vi "va-cam0#B1A2.vi"(0 "Image In":T2, 1 "Image Dst":T2, 2 "ROI Descriptor (Cent)":T1={"Global Rectangle"=[1001, 801, 1479, 1278], "Contours"=[{"ID"=enum."External", "Type"=7, "Coordinates"=[1239, 1039, 28, 238, 0, 0]}]} {"Contours"."Type" items=["No Selection", "Point", "Line", "Rectangle", "Oval", "Polygon", "Freehand Region", "Annulus", "Unused2", "Unused3", "Broken Line", "Freehand Line", "Rotated Rectangle"]}, 3 "ROI Descriptor (cir_pro_raw)":T1={"Global Rectangle"=[1854, 674, 1995, 880], "Contours"=[{"ID"=enum."External", "Type"=7, "Coordinates"=[1997, 735, 91, 143, 155136, 267537]}]} {"Contours"."Type" items=["No Selection", "Point", "Line", "Rectangle", "Oval", "Polygon", "Freehand Region", "Annulus", "Unused2", "Unused3", "Broken Line", "Freehand Line", "Rotated Rectangle"]}, 7 "error in":errorcluster) -> (19 "Caliper Results (angle_Cent_pro_fine)":sgl[][](array[numeric]) format="%.2f", 20 "Image Out":T2, 21 "Fitted Circle (Cent)":T4 {"Average SNR (dB)" format="%.2f"; "Average Strength" format="%.2f"; "Roundness (Real-World)" format="%.2f"; "Radius (Real-World)" format="%.2f"; "Center (Real-World)"."Y" format="%.2f"; "Center (Real-World)"."X" format="%.2f"; "Radius (Pixels)" format="%.2f"; "Center (Pixels)"."Y" format="%.2f"; "Center (Pixels)"."X" format="%.2f"}, 22 "Fitted Circle (cir_pro_Fine)":T4 {"Average SNR (dB)" format="%.2f"; "Average Strength" format="%.2f"; "Roundness (Real-World)" format="%.2f"; "Radius (Real-World)" format="%.2f"; "Center (Real-World)"."Y" format="%.2f"; "Center (Real-World)"."X" format="%.2f"; "Radius (Pixels)" format="%.2f"; "Center (Pixels)"."Y" format="%.2f"; "Center (Pixels)"."X" format="%.2f"}, 23 "Edge Information (edge_Find_SlotSidesLo)":T3[](array[typedef]) {"Distance (Real-World)" format="%.2f"; "Location (Real-World)"."Y" format="%.2g"; "Location (Real-World)"."X" format="%.2f"; "Noise" format="%.2f"; "Location (Pixel)"."Y" format="%.2g"; "Location (Pixel)"."X" format="%.2f"; "Strength" format="%.2f"; "Distance (Pixel)" format="%.2f"}, 26 "Edge Information (edge_Find_SlotSidesHi)":T3[](array[typedef]) {"Distance (Real-World)" format="%.2f"; "Location (Real-World)"."Y" format="%.2g"; "Location (Real-World)"."X" format="%.2f"; "Noise" format="%.2f"; "Location (Pixel)"."Y" format="%.2g"; "Location (Pixel)"."X" format="%.2f"; "Strength" format="%.2f"; "Distance (Pixel)" format="%.2f"}, 27 "error out":errorcluster)   [LabVIEW 2018]
doc: "Creates, edits, and runs vision algorithms using NI Vision Assistant.\n\nWhen you place this Express VI on the block diagram, NI Vision Assistant launches. Create an algorithm using the Vision Assistant processing functions. After you create an algorithm, you can select the controls and indicators that you want to be able to programmatically set in LabVIEW. Double-click the Vision Assistant Express VI to edit the algorithm."
uses:
  <vilib>/vision/Image Controls.llb/IMAQ Image.ctl
  <vilib>/vision/Measure.llb/Edge New.ctl
  <vilib>/vision/Measure.llb/Edge Options.ctl
  <vilib>/vision/Measure.llb/Edge Polarity.ctl
  <vilib>/vision/NI_Vision_Development_Module.lvlib
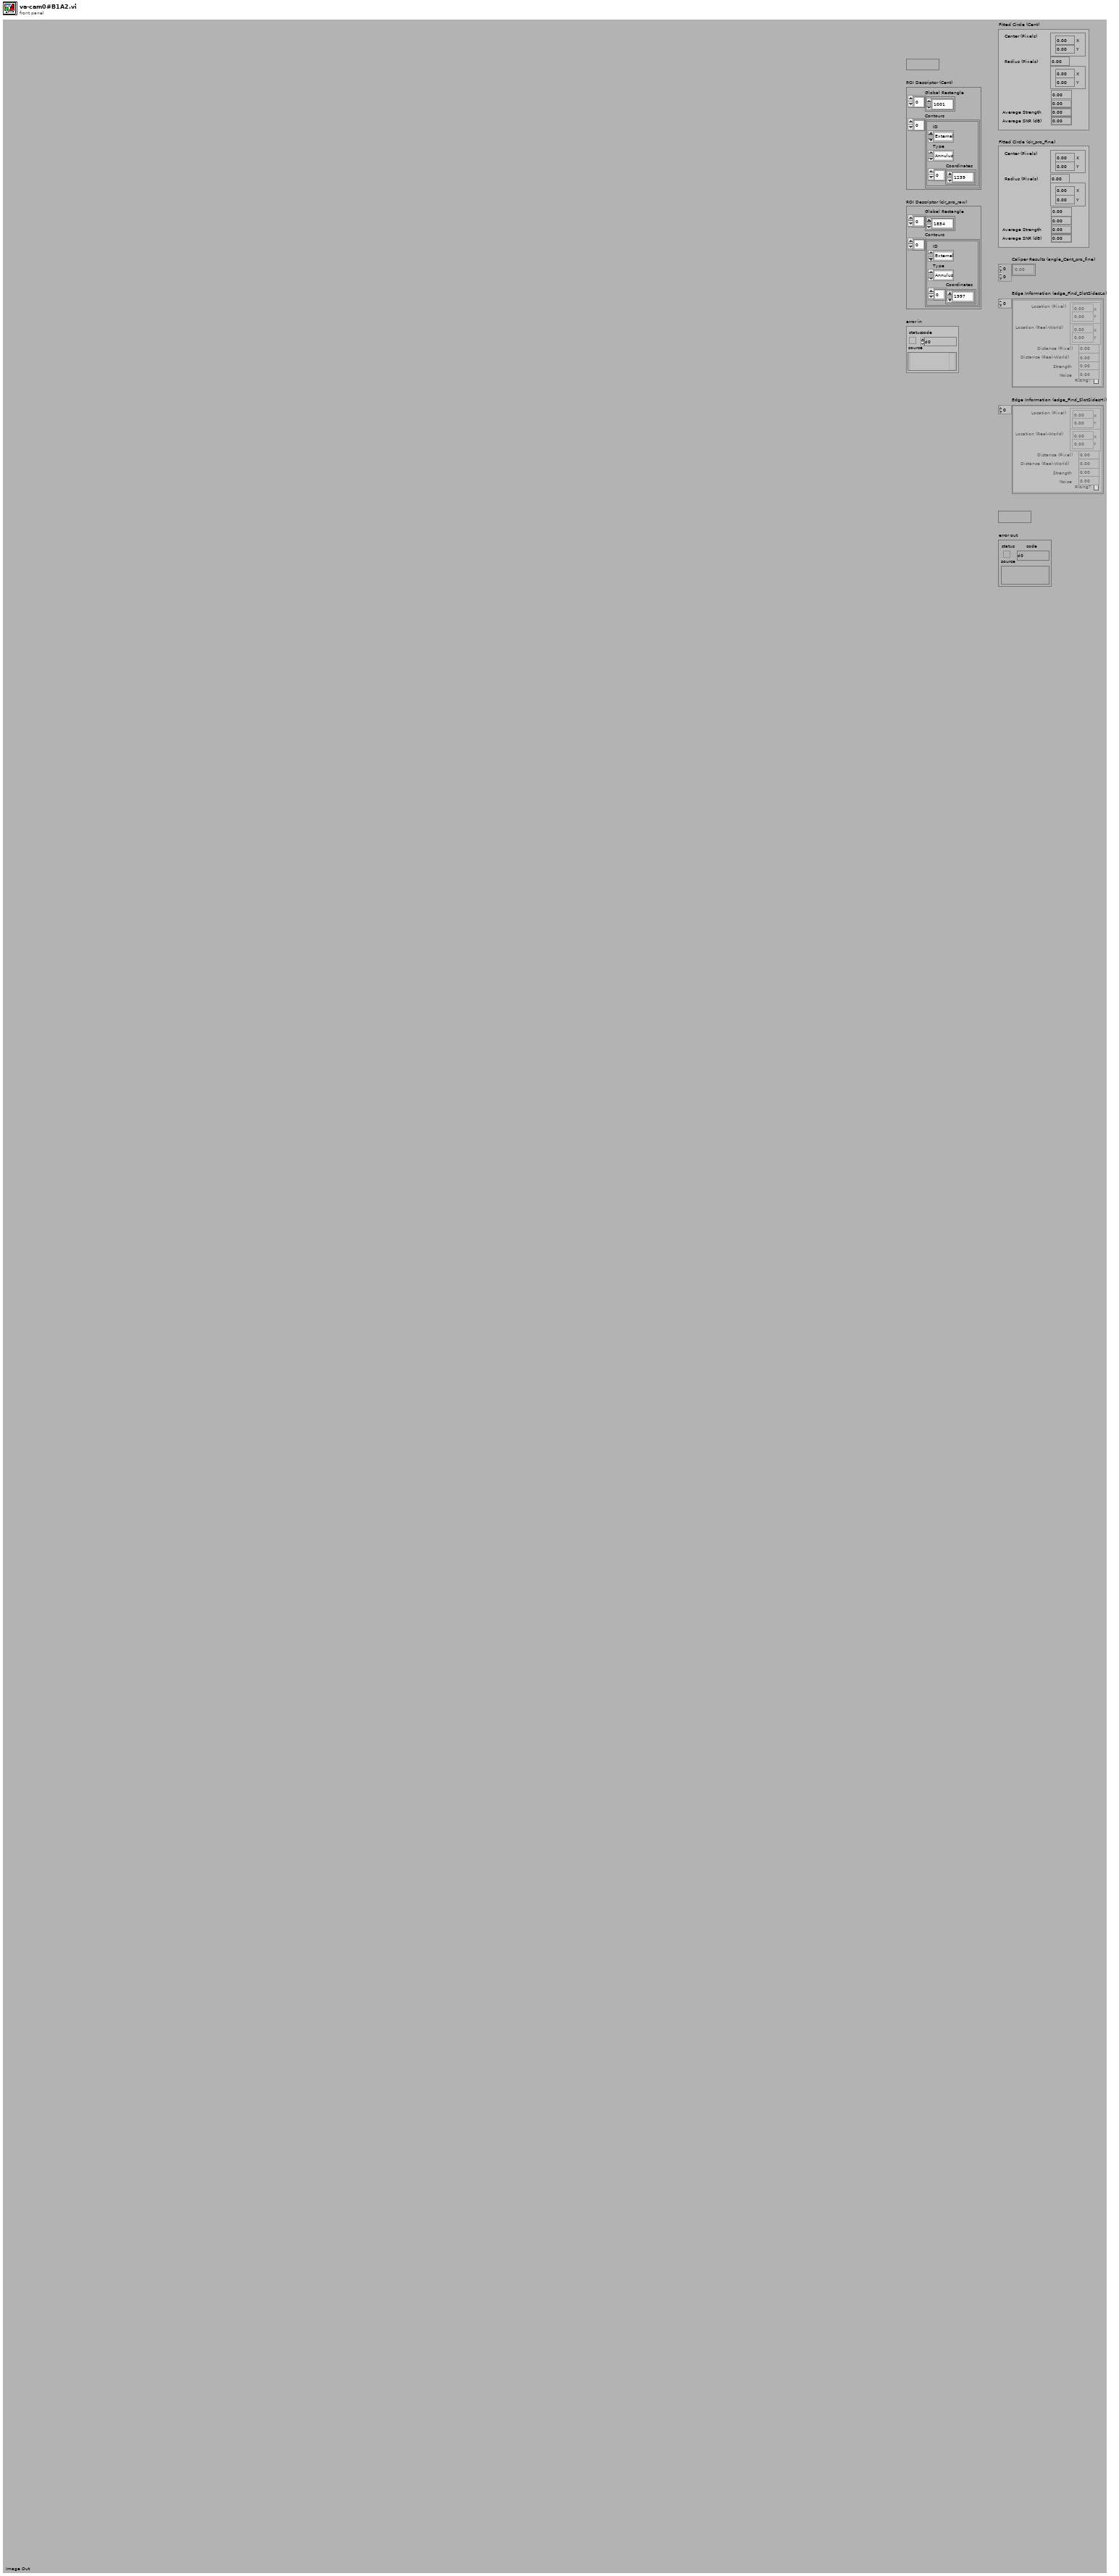
[diagram p1: front panel]
types:
  T1 = cluster{"Global Rectangle":i32[], "Contours":cluster{"ID":enum32{"External", "Internal"}, "Type":u32, "Coordinates":i32[]}[]}
  T2 = typedef "IMAQ Image.ctl" = refnum<image>
  T3 = typedef "Edge New.ctl" = cluster{"Location (Pixel)":cluster{"X":sgl, "Y":sgl}, "Location (Real-World)":cluster{"X":sgl, "Y":sgl}, "Distance (Pixel)":dbl, "Distance (Real-World)":dbl, "Strength":dbl, "Noise":dbl, "Rising?":bool}
  T4 = cluster{"Center (Pixels)":cluster{"X":sgl, "Y":sgl}, "Radius (Pixels)":dbl, "Center (Real-World)":cluster{"X":sgl, "Y":sgl}, "Radius (Real-World)":dbl, "Roundness (Real-World)":dbl, "Average Strength":dbl, "Average SNR (dB)":dbl}
  T5 = cluster{"Edge Polarity":u32, "Kernel Size":u32, "Width":u32, "Minimum Edge Strength":sgl, "Interpolation Type":enum32{"Zero Order", "Bilinear", "Quadratic", "Cubic", "Bilinear Fixed"}, "Data Processing Method":enum32{"Average", "Median"}}
  T6 = enum16{"Get First Edge", "Get First + Last Edge", "Get All Edges", "Get Best Edge"}
  T7 = cluster{"Origin":cluster{"X":sgl, "Y":sgl}, "Angle (deg)":sgl, "Axis Reference":u32}
  T8 = enum16{"Reset", "Update Coordinate System", "Get Coordinate System"}
  T9 = enum16{"Horizontal Motion", "Vertical Motion", "Horizontal and Vertical Motion", "Horizontal, Vertical and Angular Motion"}
  T10 = cluster{"Feature":u32, "Points IDs":cluster{"GUID":string, "Index":i32}[]}[]
  T11 = typedef "Edge Options.ctl" = cluster{"Edge Polarity":T12, "Kernel Size":u32, "Width":u32, "Minimum Edge Strength":sgl, "Interpolation Type":enum32{"Zero Order", "Bilinear", "Quadratic", "Cubic", "Bilinear Fixed"}, "Data Processing Method":enum32{"Average", "Median"}}
  T12 = typedef "Edge Polarity.ctl" = u32
  T13 = cluster{"Search  Direction":u32, "Edge Options":T11, "Show Search Area":bool, "Show Search Lines":bool, "Show Edges Found":bool, "Show Result":bool, "Search Area Color":u32, "Search Lines Color":u32, "Edge Locations Color":u32, "Result Color":u32, "Overlay Group Name":string}
  T14 = cluster{"Process":enum16{"Get First Edge", "Get First + Last Edge", "Get All Edges", "Get Best Edge"}, "Step Size":i32, "Max Pixel Radius":i32}
  T15 = typedef "Image Type" = u32
  T16 = typedef "IMAQ Coordinate System" = cluster{"Reference System":cluster{"Origin":cluster{"X":sgl, "Y":sgl}, "Angle (deg)":sgl, "Axis Reference":u32}, "Measurement System":cluster{"Origin":cluster{"X":sgl, "Y":sgl}, "Angle (deg)":sgl, "Axis Reference":u32}}
  T17 = typedef "ROI Descriptor" = cluster{"Global Rectangle":i32[], "Contours":cluster{"ID":enum32{"External", "Internal"}, "Type":u32, "Coordinates":i32[]}[]}
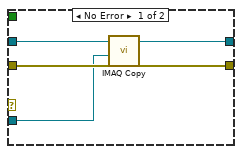
[diagram p10: hidden frame]
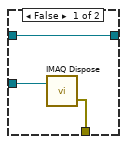
[diagram p12: hidden frame]
diagram:
  w105 = T15 4 items=["Grayscale (U8)", "Grayscale (I16)", "Grayscale (SGL)", "Complex (CSG)", "RGB (U32)", "HSL (U32)", "RGB (U64)", "Grayscale (U16)"] ("Image Dst Type")
  w106 = T15 4 items=["Grayscale (U8)", "Grayscale (I16)", "Grayscale (SGL)", "Complex (CSG)", "RGB (U32)", "HSL (U32)", "RGB (U64)", "Grayscale (U16)"] ("Image Type")
  w125 = TRUE  # Backup Copy
  w118 = FALSE  # Create Image Dst
  # "Caliper"
  # "Caliper"
  n1 = Call Chain() -> (call chain=w112:string[])
  n2 = Index Array(array=w112) -> (element=w111:string)  [unwired: 1 in]
  n3 = Concatenate Strings("20202189 Backup" ("Backup Image Name"), " ", w111) -> (w108:string)
  n4 = call "IMAQ Create"("Image Name"=w108, "Image Type"=w106) -> ("New Image"=w107:T2)  [unwired: 2 in, 2 out]
  n5 = case "Create backup copy for edition purposes" shown="真" w125 {
    tunnel: [w128 w131] -> w121
    tunnel: "Image In" -> [w128 w131]
    tunnel: w107 -> [w127 w130]
    tunnel: [w126 w129] -> w1
    frame False {
      n6 = call "IMAQ Dispose"("Image"=w127) -> ("error out"=w126:errorcluster)  [unwired: 2 in, 3 out]
    }
    frame True {
      n7 = call "IMAQ Copy"("Image Dst"=w130, "Image Src"=w131) -> ("error out"=w129:errorcluster)  [unwired: 1 in, 4 out]
    }
  }
  n8 = call <vilib>:"Clear Errors.vi"("error in (no error)"=w1) -> ()  [unwired: 5 in, 2 out]
  n9 = Call Chain() -> (call chain=w117:string[])
  n10 = call "IMAQ GetImageInfo"("Image"="Image Dst") -> ("error out"=w123:errorcluster)  [unwired: 1 in, 9 out]
  n11 = Index Array(array=w117) -> (element=w115:string)  [unwired: 1 in]
  n12 = Concatenate Strings("20202189 Dst" ("Image Dst Name"), " ", w115) -> (w113:string)
  n13 = case "条件结构" shown="错误" w123 {
    tunnel: [w136 w140] -> w104
    tunnel: [w135 w139] -> w119
    tunnel: w121 -> [w134 w141]
    tunnel: "error in" -> [w133 w137]
    tunnel: "Image Dst" -> [w132 _]
    tunnel: w113 -> [_ w143]
    tunnel: w105 -> [_ w142]
    tunnel: w118 -> [_ w138]
    frame No Error {
      n14 = call "IMAQ Copy"("error in (no error)"=w133, "Image Dst"=w132, "Image Src"=w134) -> ("error out"=w135:errorcluster, "Image Dst Out"=w136:T2)  [unwired: 3 out]
    }
    frame Error {
      n15 = case "条件结构" shown="真" w138 {
        tunnel: w143 -> [_ w152]
        tunnel: w142 -> [_ w151]
        tunnel: w141 -> [w145 w149]
        tunnel: [w145 w148] -> w140
        tunnel: [w144 w147] -> w139
        tunnel: w137 -> [w144 _]
        frame False {
        }
        frame True {
          n16 = call "IMAQ Create"("Image Name"=w152, "Image Type"=w151) -> ("New Image"=w150:T2, "error out"=w146:errorcluster)  [unwired: 2 in, 1 out]
          n17 = call "IMAQ Copy"("error in (no error)"=w146, "Image Dst"=w150, "Image Src"=w149) -> ("error out"=w147:errorcluster, "Image Dst Out"=w148:T2)  [unwired: 3 out]
        }
      }
    }
  }
  n18 = Unbundle By Name(w119) -> ("code"=w100:i32)
  n19 = case "条件结构" shown="默认" w100 {
    tunnel: T13 {"Search  Direction"=0, "Edge Options"={"Edge Polarity"=2, "Kernel Size"=9, "Width"=3, "Minimum Edge Strength"=80.0, "Interpolation Type"=enum."Bilinear Fixed", "Data Processing Method"=enum."Average"}, "Show Search Area"=TRUE, "Show Search Lines"=TRUE, "Show Edges Found"=TRUE, "Show Result"=TRUE, "Search Area Color"=65280, "Search Lines Color"=255, "Edge Locations Color"=16776960, "Result Color"=16711680, "Overlay Group Name"=""} ("Options") -> [_ w154]
    tunnel: w104 -> [w153 w164]
    tunnel: w119 -> [_ w163]
    tunnel: [_ w161] -> w103
    tunnel: [w153 w159] -> w89
    tunnel: "Cent" ("Step Name") -> [_ w158]
    tunnel: "ROI Descriptor (Cent)" -> [_ w157]
    tunnel: T14 {"Process"=enum."Get First Edge", "Step Size"=15, "Max Pixel Radius"=3} ("Circle Fit Options") -> [_ w156]
    tunnel: [_ w155] -> w98
    frame -1074396199, -1074396198 {
      # "Discard Coordinate System Error"
    }
    frame Default {
      n20 = call "IMAQ Find Circular Edge 3"("Circle Fit Options"=w156, "Options"=w154, "error in (no error)"=w163, "ROI Descriptor"=w157, "Image"=w164) -> ("error out"=w162:errorcluster, "Fitted Circle"=w155:T4, "Image Out"=w160:T2)  [unwired: 2 in, 2 out]
      n21 = call <vilib>:"IVA Store Circular Edge2 Results.vi"("error in (no error)"=w162, "Step Name"=w158, "Fitted Circle"=w155, "Image in"=w160) -> ("error out"=w161:errorcluster, "Image dup"=w159:T2)  [unwired: 2 in, 4 out]
    }
  }
  "Fitted Circle (Cent)" <- w98
  n22 = call <vilib>:"IVA Coordinate System Manager 2.vi"("Mode"=T9."Horizontal and Vertical Motion", "Reference System"=T7 {"Origin"={"X"=948.91205, "Y"=610.65265}, "Angle (deg)"=0.0, "Axis Reference"=0}, "Function"=T8."Update Coordinate System", "error in (no error)"=w103, "Angle ID"=cluster{"GUID":string, "Index":i32} {"GUID"="", "Index"=0}, "Origin ID"=cluster{"GUID":string, "Index":i32} {"GUID"="Cent", "Index"=0}, "Coordinate System Name"="co_cent") -> ("error out"=w90:errorcluster)  [unwired: 4 out]
  n23 = Unbundle By Name(w90) -> ("code"=w85:i32)
  n24 = case "条件结构" shown="默认" w85 {
    tunnel: T13 {"Search  Direction"=0, "Edge Options"={"Edge Polarity"=2, "Kernel Size"=11, "Width"=13, "Minimum Edge Strength"=50.0, "Interpolation Type"=enum."Bilinear Fixed", "Data Processing Method"=enum."Average"}, "Show Search Area"=TRUE, "Show Search Lines"=TRUE, "Show Edges Found"=TRUE, "Show Result"=TRUE, "Search Area Color"=65280, "Search Lines Color"=255, "Edge Locations Color"=16776960, "Result Color"=16711680, "Overlay Group Name"=""} ("Options") -> [_ w166]
    tunnel: w89 -> [w165 w176]
    tunnel: w90 -> [_ w175]
    tunnel: [_ w173] -> w88
    tunnel: [w165 w171] -> w82
    tunnel: "cir_pro_raw" ("Step Name") -> [_ w170]
    tunnel: "ROI Descriptor (cir_pro_raw)" -> [_ w169]
    tunnel: T14 {"Process"=enum."Get First Edge", "Step Size"=10, "Max Pixel Radius"=3} ("Circle Fit Options") -> [_ w168]
    tunnel: [_ w167] -> _
    frame -1074396199, -1074396198 {
      # "Discard Coordinate System Error"
    }
    frame Default {
      n25 = call "IMAQ Find Circular Edge 3"("Circle Fit Options"=w168, "Options"=w166, "error in (no error)"=w175, "ROI Descriptor"=w169, "Image"=w176) -> ("error out"=w174:errorcluster, "Fitted Circle"=w167:T4, "Image Out"=w172:T2)  [unwired: 2 in, 2 out]
      n26 = call <vilib>:"IVA Store Circular Edge2 Results.vi"("error in (no error)"=w174, "Step Name"=w170, "Fitted Circle"=w167, "Image in"=w172) -> ("error out"=w173:errorcluster, "Image dup"=w171:T2)  [unwired: 2 in, 4 out]
    }
  }
  n27 = call <vilib>:"IVA Caliper Sub-VI 3.vi"("error in"=w88, "Parameters"=T10 [{"Feature"=4, "Points IDs"=[{"GUID"="Cent", "Index"=0}, {"GUID"="cir_pro_raw", "Index"=0}]}], "Step Name"="angle_Cent2Pro_raw", "Image In"=w82) -> ("error out"=w81:errorcluster, "Image Out"=w62:T2)  [unwired: 1 in, 5 out]
  n28 = call <vilib>:"IVA Coordinate System Manager 2.vi"("Mode"=T9."Horizontal, Vertical and Angular Motion", "Reference System"=T7 {"Origin"={"X"=1204.4635, "Y"=165.70685}, "Angle (deg)"=60.573715, "Axis Reference"=0}, "Function"=T8."Update Coordinate System", "error in (no error)"=w81, "Angle ID"=cluster{"GUID":string, "Index":i32} {"GUID"="angle_Cent2Pro_raw", "Index"=0}, "Origin ID"=cluster{"GUID":string, "Index":i32} {"GUID"="cir_pro_raw", "Index"=0}, "Coordinate System Name"="co_pro_Raw") -> ("error out"=w72:errorcluster)  [unwired: 4 out]
  n29 = call <vilib>:"IVA Coordinate System Manager 2.vi"("Reference System"=T7 {"Origin"={"X"=1991.2946, "Y"=743.0359}, "Angle (deg)"=21.639477, "Axis Reference"=0}, "Function"=T8."Get Coordinate System", "error in (no error)"=w72, "Coordinate System Name"="co_pro_Raw") -> ("error out"=w69:errorcluster, "Coordinate System Out"=w65:T16)  [unwired: 3 in, 3 out]
  n30 = call <vilib>:"IVA Check Coordinate System Valid 2.vi"("error in (no error)"=w69, "Coordinate System"=w65) -> ("error out"=w63:errorcluster, "Valid?"=w64:bool)  [unwired: 8 out]
  n31 = case "条件结构" shown="真" w64 {
    tunnel: T1 {"Global Rectangle"=[1831, 643, 1989, 904], "Contours"=[{"ID"=enum."External", "Type"=7, "Coordinates"=[1989, 744, 51, 158, 140548, 267955]}]} ("ROI Descriptor") -> [w178 w185]
    tunnel: [w178 w182] -> w59
    tunnel: [w177 w181] -> w66
    tunnel: w65 -> [_ w180]
    tunnel: w63 -> [w177 w179]
    frame False {
    }
    frame True {
      n32 = Unbundle By Name(w180) -> ("Reference System"=w184:T7, "Measurement System"=w183:T7)
      n33 = call "IMAQ TransformROI"("error in (no error)"=w179, "New Reference"=w183, "Base Reference"=w184, "ROI Descriptor"=w185) -> ("error out"=w181:errorcluster, "ROI Descriptor out"=w182:T17)  [unwired: 6 out]
    }
  }
  n34 = Unbundle By Name(w66) -> ("code"=w58:i32)
  n35 = case "条件结构" shown="默认" w58 {
    tunnel: T13 {"Search  Direction"=1, "Edge Options"={"Edge Polarity"=1, "Kernel Size"=13, "Width"=13, "Minimum Edge Strength"=50.0, "Interpolation Type"=enum."Bilinear Fixed", "Data Processing Method"=enum."Average"}, "Show Search Area"=TRUE, "Show Search Lines"=TRUE, "Show Edges Found"=TRUE, "Show Result"=TRUE, "Search Area Color"=65280, "Search Lines Color"=255, "Edge Locations Color"=16776960, "Result Color"=16711680, "Overlay Group Name"=""} ("Options") -> [_ w187]
    tunnel: w62 -> [w186 w197]
    tunnel: w66 -> [_ w196]
    tunnel: [_ w194] -> w61
    tunnel: [w186 w192] -> w54
    tunnel: "cir_pro_Fine" ("Step Name") -> [_ w191]
    tunnel: w59 -> [_ w190]
    tunnel: T14 {"Process"=enum."Get First Edge", "Step Size"=10, "Max Pixel Radius"=3} ("Circle Fit Options") -> [_ w189]
    tunnel: [_ w188] -> w56
    frame -1074396199, -1074396198 {
      # "Discard Coordinate System Error"
    }
    frame Default {
      n36 = call "IMAQ Find Circular Edge 3"("Circle Fit Options"=w189, "Options"=w187, "error in (no error)"=w196, "ROI Descriptor"=w190, "Image"=w197) -> ("error out"=w195:errorcluster, "Fitted Circle"=w188:T4, "Image Out"=w193:T2)  [unwired: 2 in, 2 out]
      n37 = call <vilib>:"IVA Store Circular Edge2 Results.vi"("error in (no error)"=w195, "Step Name"=w191, "Fitted Circle"=w188, "Image in"=w193) -> ("error out"=w194:errorcluster, "Image dup"=w192:T2)  [unwired: 2 in, 4 out]
    }
  }
  "Fitted Circle (cir_pro_Fine)" <- w56
  n38 = call <vilib>:"IVA Caliper Sub-VI 3.vi"("error in"=w61, "Parameters"=T10 [{"Feature"=4, "Points IDs"=[{"GUID"="Cent", "Index"=0}, {"GUID"="cir_pro_Fine", "Index"=0}]}], "Step Name"="angle_Cent_pro_fine", "Image In"=w54) -> ("error out"=w53:errorcluster, "Results (Pixels)"=→"Caliper Results (angle_Cent_pro_fine)":sgl[][], "Image Out"=w33:T2)  [unwired: 1 in, 4 out]
  n39 = call <vilib>:"IVA Coordinate System Manager 2.vi"("Mode"=T9."Horizontal, Vertical and Angular Motion", "Reference System"=T7 {"Origin"={"X"=1200.5801, "Y"=172.7976}, "Angle (deg)"=60.72441, "Axis Reference"=0}, "Function"=T8."Update Coordinate System", "error in (no error)"=w53, "Angle ID"=cluster{"GUID":string, "Index":i32} {"GUID"="angle_Cent_pro_fine", "Index"=0}, "Origin ID"=cluster{"GUID":string, "Index":i32} {"GUID"="cir_pro_Fine", "Index"=0}, "Coordinate System Name"="co_pro_Fine") -> ("error out"=w43:errorcluster)  [unwired: 4 out]
  n40 = call <vilib>:"IVA Coordinate System Manager 2.vi"("Reference System"=T7 {"Origin"={"X"=1991.6995, "Y"=743.72284}, "Angle (deg)"=21.583755, "Axis Reference"=0}, "Function"=T8."Get Coordinate System", "error in (no error)"=w43, "Coordinate System Name"="co_pro_Fine") -> ("error out"=w40:errorcluster, "Coordinate System Out"=w36:T16)  [unwired: 3 in, 3 out]
  n41 = call <vilib>:"IVA Check Coordinate System Valid 2.vi"("error in (no error)"=w40, "Coordinate System"=w36) -> ("error out"=w34:errorcluster, "Valid?"=w35:bool)  [unwired: 8 out]
  n42 = case "条件结构" shown="真" w35 {
    tunnel: T1 {"Global Rectangle"=[1911, 698, 1966, 836], "Contours"=[{"ID"=enum."External", "Type"=2, "Coordinates"=[1911, 698, 1965, 835]}]} ("ROI Descriptor") -> [w199 w206]
    tunnel: [w199 w203] -> w24
    tunnel: [w198 w202] -> w37
    tunnel: w36 -> [_ w201]
    tunnel: w34 -> [w198 w200]
    frame False {
    }
    frame True {
      n43 = Unbundle By Name(w201) -> ("Reference System"=w205:T7, "Measurement System"=w204:T7)
      n44 = call "IMAQ TransformROI"("error in (no error)"=w200, "New Reference"=w204, "Base Reference"=w205, "ROI Descriptor"=w206) -> ("error out"=w202:errorcluster, "ROI Descriptor out"=w203:T17)  [unwired: 6 out]
    }
  }
  n45 = Unbundle By Name(w37) -> ("code"=w23:i32)
  n46 = case "条件结构" shown="默认" w23 {
    tunnel: w37 -> [_ w217]
    tunnel: w33 -> [w207 w216]
    tunnel: T6."Get All Edges" ("Process") -> [_ w215]
    tunnel: T5 {"Edge Polarity"=0, "Kernel Size"=3, "Width"=25, "Minimum Edge Strength"=20.0, "Interpolation Type"=enum."Bilinear Fixed", "Data Processing Method"=enum."Average"} ("Edge Options") -> [_ w214]
    tunnel: [_ w213] -> w30
    tunnel: [w207 w212] -> w28
    tunnel: [_ w211] -> w27
    tunnel: w24 -> [_ w210]
    frame -1074396199, -1074396198 {
    }
    frame Default {
      n47 = call "IMAQ Edge Tool 3"("Image"=w216, "Edge Options"=w214, "Optimized Mode"=TRUE, "ROI Descriptor"=w210, "Process"=w215, "error in (no error)"=w217, "Reverse Direction"=FALSE) -> ("Image (duplicate)"=w212:T2, "Edge Information"=w211:T3[], "error out"=w213:errorcluster)  [unwired: 6 out]
    }
  }
  n48 = call <vilib>:"IVA Store Advanced Edges Results.vi"("error in (no error)"=w30, "Step Name"="edge_Find_SlotSidesLo", "Edge Information"=w27, "Image in"=w28) -> ("error out"=w29:errorcluster, "Edge Information dup"=→"Edge Information (edge_Find_SlotSidesLo)":T3[], "Image dup"=w13:T2)  [unwired: 5 out]
  n49 = call <vilib>:"IVA Coordinate System Manager 2.vi"("Reference System"=T7 {"Origin"={"X"=1991.6995, "Y"=743.72284}, "Angle (deg)"=21.583755, "Axis Reference"=0}, "Function"=T8."Get Coordinate System", "error in (no error)"=w29, "Coordinate System Name"="co_pro_Fine") -> ("error out"=w20:errorcluster, "Coordinate System Out"=w16:T16)  [unwired: 3 in, 3 out]
  n50 = call <vilib>:"IVA Check Coordinate System Valid 2.vi"("error in (no error)"=w20, "Coordinate System"=w16) -> ("error out"=w14:errorcluster, "Valid?"=w15:bool)  [unwired: 8 out]
  n51 = case "条件结构" shown="真" w15 {
    tunnel: T1 {"Global Rectangle"=[1927, 691, 1984, 829], "Contours"=[{"ID"=enum."External", "Type"=2, "Coordinates"=[1927, 691, 1983, 828]}]} ("ROI Descriptor") -> [w219 w226]
    tunnel: [w219 w223] -> w4
    tunnel: [w218 w222] -> w17
    tunnel: w16 -> [_ w221]
    tunnel: w14 -> [w218 w220]
    frame False {
    }
    frame True {
      n52 = Unbundle By Name(w221) -> ("Reference System"=w225:T7, "Measurement System"=w224:T7)
      n53 = call "IMAQ TransformROI"("error in (no error)"=w220, "New Reference"=w224, "Base Reference"=w225, "ROI Descriptor"=w226) -> ("error out"=w222:errorcluster, "ROI Descriptor out"=w223:T17)  [unwired: 6 out]
    }
  }
  n54 = Unbundle By Name(w17) -> ("code"=w3:i32)
  n55 = case "条件结构" shown="默认" w3 {
    tunnel: w17 -> [_ w237]
    tunnel: w13 -> [w227 w236]
    tunnel: T6."Get All Edges" ("Process") -> [_ w235]
    tunnel: T5 {"Edge Polarity"=0, "Kernel Size"=3, "Width"=25, "Minimum Edge Strength"=20.0, "Interpolation Type"=enum."Bilinear Fixed", "Data Processing Method"=enum."Average"} ("Edge Options") -> [_ w234]
    tunnel: [_ w233] -> w10
    tunnel: [w227 w232] -> w8
    tunnel: [_ w231] -> w7
    tunnel: w4 -> [_ w230]
    frame -1074396199, -1074396198 {
    }
    frame Default {
      n56 = call "IMAQ Edge Tool 3"("Image"=w236, "Edge Options"=w234, "Optimized Mode"=TRUE, "ROI Descriptor"=w230, "Process"=w235, "error in (no error)"=w237, "Reverse Direction"=FALSE) -> ("Image (duplicate)"=w232:T2, "Edge Information"=w231:T3[], "error out"=w233:errorcluster)  [unwired: 6 out]
    }
  }
  n57 = call <vilib>:"IVA Store Advanced Edges Results.vi"("error in (no error)"=w10, "Step Name"="edge_Find_SlotSidesHi", "Edge Information"=w7, "Image in"=w8) -> ("error out"=→"error out":errorcluster, "Edge Information dup"=→"Edge Information (edge_Find_SlotSidesHi)":T3[], "Image dup"=→"Image Out":T2)  [unwired: 5 out]
